vi "AquireTape.vi"(8 "error in (no error)":errorcluster, 10 "Settings":T1={"max velocity"={"Value"=0.0, "Min"=0.0, "Max"=0.0, "StepSize"=0.0, "Tolerance"=0.0, "ValueActual"=0.0}, "continious velocity"={"Value"=0.0, "Min"=0.0, "Max"=0.0, "StepSize"=0.0, "Tolerance"=0.0, "ValueActual"=0.0}, "shake"=enum."off", "direction"=enum."left", "RedRatio"={"Value"=0.0, "Min"=0.0, "Max"=0.0, "StepSize"=0.0, "Tolerance"=0.0, "ValueActual"=0.0}, "StepSize"={"Value"=0.0, "Min"=0.0, "Max"=0.0, "StepSize"=0.0, "Tolerance"=0.0, "ValueActual"=0.0}, "position"={"Value"=0.0, "Min"=0.0, "Max"=0.0, "StepSize"=0.0, "Tolerance"=0.0, "ValueActual"=0.0}, "velocity"={"Value"=0.0, "Min"=0.0, "Max"=0.0, "StepSize"=0.0, "Tolerance"=0.0, "ValueActual"=0.0}, "Step"=enum."off", "Mode"=enum."on demand", "timeout"={"Value"=0.0, "Min"=0.0, "Max"=0.0, "StepSize"=0.0, "Tolerance"=0.0, "ValueActual"=0.0}, "DelayStage"={"Value"=0.0, "Min"=0.0, "Max"=0.0, "StepSize"=0.0, "Tolerance"=0.0, "ValueActual"=0.0}, "TapeMotor"=enum."off", "encoder Axis"=2, "oldpos"=0.0, "ResetEncoder"=enum."off", "tape monitor"=enum."off", "ComPort"="COM1", "Stream Settings"={"My Name"="TapeDrive", "Remote IP Address"="localhost", "Remote Name"="RT"}, "Motor1Axis"={"Value"=0.0, "Min"=0.0, "Max"=0.0, "StepSize"=0.0, "Tolerance"=0.0, "ValueActual"=0.0}, "Motor2Axis"={"Value"=0.0, "Min"=0.0, "Max"=0.0, "StepSize"=0.0, "Tolerance"=0.0, "ValueActual"=0.0}}, 11 "VISA Refnum in":refnum<visa-resource-name>) -> (0 "error out":errorcluster, 1 "RedRatio":dbl, 2 "Settings":T1={"max velocity"={"Value"=0.0, "Min"=0.0, "Max"=0.0, "StepSize"=0.0, "Tolerance"=0.0, "ValueActual"=0.0}, "continious velocity"={"Value"=0.0, "Min"=0.0, "Max"=0.0, "StepSize"=0.0, "Tolerance"=0.0, "ValueActual"=0.0}, "shake"=enum."off", "direction"=enum."left", "RedRatio"={"Value"=0.0, "Min"=0.0, "Max"=0.0, "StepSize"=0.0, "Tolerance"=0.0, "ValueActual"=0.0}, "StepSize"={"Value"=0.0, "Min"=0.0, "Max"=0.0, "StepSize"=0.0, "Tolerance"=0.0, "ValueActual"=0.0}, "position"={"Value"=0.0, "Min"=0.0, "Max"=0.0, "StepSize"=0.0, "Tolerance"=0.0, "ValueActual"=0.0}, "velocity"={"Value"=0.0, "Min"=0.0, "Max"=0.0, "StepSize"=0.0, "Tolerance"=0.0, "ValueActual"=0.0}, "Step"=enum."off", "Mode"=enum."on demand", "timeout"={"Value"=0.0, "Min"=0.0, "Max"=0.0, "StepSize"=0.0, "Tolerance"=0.0, "ValueActual"=0.0}, "DelayStage"={"Value"=0.0, "Min"=0.0, "Max"=0.0, "StepSize"=0.0, "Tolerance"=0.0, "ValueActual"=0.0}, "TapeMotor"=enum."off", "encoder Axis"=2, "oldpos"=0.0, "ResetEncoder"=enum."off", "tape monitor"=enum."off", "ComPort"="COM1", "Stream Settings"={"My Name"="TapeDrive", "Remote IP Address"="localhost", "Remote Name"="RT"}, "Motor1Axis"={"Value"=0.0, "Min"=0.0, "Max"=0.0, "StepSize"=0.0, "Tolerance"=0.0, "ValueActual"=0.0}, "Motor2Axis"={"Value"=0.0, "Min"=0.0, "Max"=0.0, "StepSize"=0.0, "Tolerance"=0.0, "ValueActual"=0.0}}, 3 "VISA Refnum out":refnum<visa-resource-name>, 4 "Position (units)":dbl, 6 "velocity":dbl)   [LabVIEW 2020]
uses:
  settings_TypDef.ctl
  shared/numericVariable_TypeDef.ctl
  shared/OnOffTypeDef.ctl
  Direction_TypDef.ctl
  Mode_TypDEf.ctl
  <vilib>/addons/_JKI.lib/Network_Streams_Connection.llb/PublicSettings.ctl
  shared/CompressAndUpdate(Poly)/CompressAndUpdate(Numeric).vi
  Newport ESP301/Newport ESP301.lvlib
  BaseDriver/BaseDriver.lvclass
  TapeDrive.lvclass
  <vilib>/addons/_JKI.lib/Network_Streams_Connection.llb/NetworkConnection.lvclass
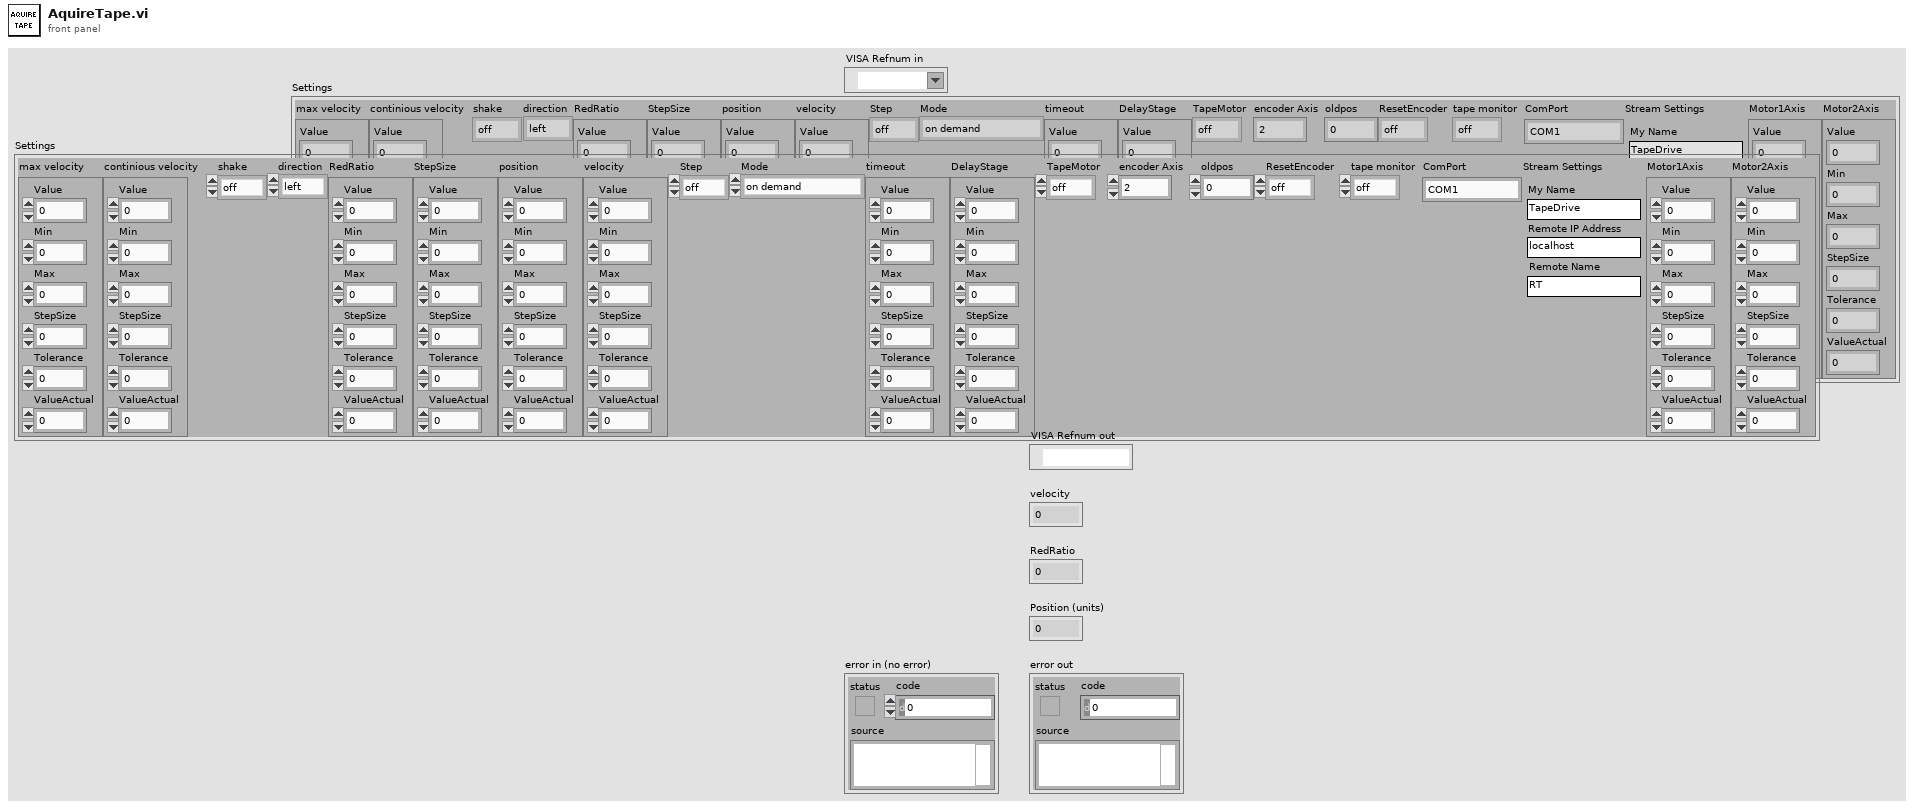
[diagram p1: front panel]
types:
  T1 = typedef "TapeDrive.lvclass/settings_TypDef.ctl" = cluster{"max velocity":T2, "continious velocity":T2, "shake":T3, "direction":T4, "RedRatio":T2, "StepSize":T2, "position":T2, "velocity":T2, "Step":T3, "Mode":T5, "timeout":T2, "DelayStage":T2, "TapeMotor":T3, "encoder Axis":i32, "oldpos":dbl, "ResetEncoder":T3, "tape monitor":T3, "ComPort":string, "Stream Settings":T6, "Motor1Axis":T2, "Motor2Axis":T2}
  T2 = typedef "BaseDriver.lvclass/numericVariable_TypeDef.ctl" = cluster{"Value":dbl, "Min":dbl, "Max":dbl, "StepSize":dbl, "Tolerance":dbl, "ValueActual":dbl}
  T3 = typedef "OnOffTypeDef.ctl" = enum16{"off", "on"}
  T4 = typedef "Direction_TypDef.ctl" = enum16{"left", "right"}
  T5 = typedef "Mode_TypDEf.ctl" = enum16{"on demand", "continuous", "scan"}
  T6 = typedef "NetworkConnection.lvclass/PublicSettings.ctl" = cluster{"My Name":string, "Remote IP Address":string, "Remote Name":string}
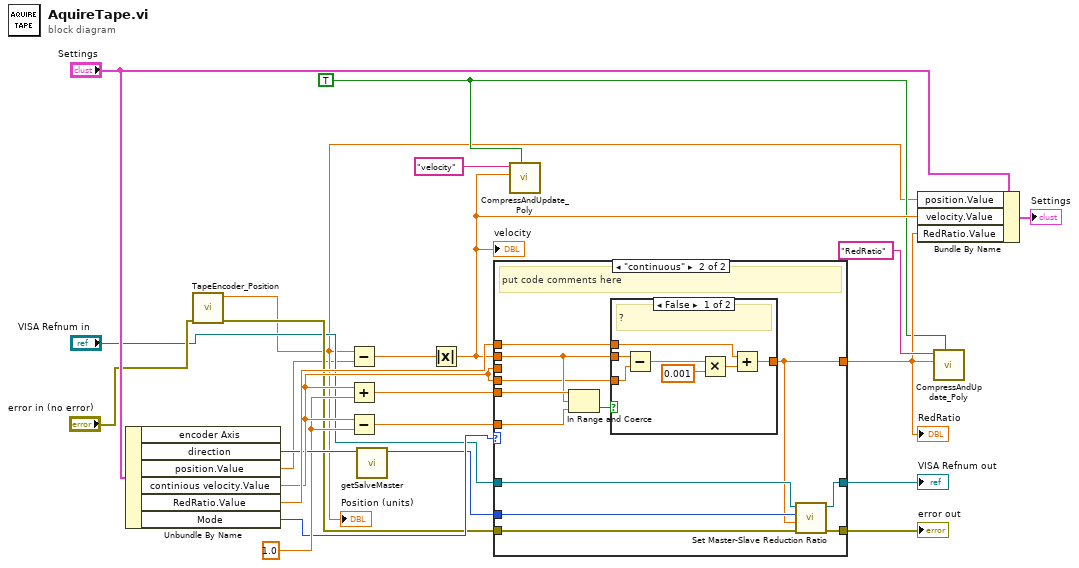
[diagram p0: block diagram]
diagram:
  w8 = TRUE ("force CVT update (false)")
  w16 = 1.0 ("y")
  n1 = Unbundle By Name("Settings") -> ("direction"=w19:T4, "position.Value"=w1:dbl, "continious velocity.Value"=w21:dbl, "RedRatio.Value"=w23:dbl, "Mode"=w7:T5)  [unwired: 1 out]
  n2 = call "TapeEncoder_Position.vi"("error in (no error)"="error in (no error)") -> ("error IO"=w4:errorcluster, "position"=w2:dbl)  [unwired: 9 in]
  "Position (units)" <- w2
  n3 = Subtract(x=w2, y=w1) -> (x-y=w13:dbl)
  n4 = Add(x=w21, y=w16) -> (x+y=w17:dbl)
  n5 = Subtract(x=w21, y=w16) -> (x-y=w18:dbl)
  n6 = call "getSalveMaster.vi"("direction"=w19) -> ("Slave"=w6:i32)  [unwired: 9 in, 1 out]
  n7 = Absolute Value(x=w13) -> (abs(x)=w11:dbl)
  "velocity" <- w11
  n8 = case shown="\"continuous\"" w7 {
    tunnel: "VISA Refnum in" -> [w26 w38]
    tunnel: [w26 w37] -> w14
    tunnel: w4 -> [w25 w36]
    tunnel: [w25 w35] -> w15
    tunnel: w6 -> [_ w34]
    tunnel: w21 -> [_ _]
    tunnel: w11 -> [_ w30]
    tunnel: w17 -> [_ w33]
    tunnel: w18 -> [_ w32]
    tunnel: w21 -> [_ w29]
    tunnel: w23 -> [w24 w28]
    tunnel: [w24 w27] -> w9
    frame "on demand", Default {
    }
    frame "continuous" {
      # "put code comments here"
      n9 = In Range and Coerce(upper limit=w33, x=w30, lower limit=w32) -> (In Range?=w31:bool)  [unwired: 1 out]
      n10 = case shown="False" w31 {
        tunnel: w30 -> [w45 _]
        tunnel: w29 -> [w44 _]
        tunnel: [w40 w46] -> w27
        tunnel: w28 -> [w39 w46]
        frame False {
          # "?"
          n11 = Subtract(x=w45, y=w44) -> (x-y=w43:dbl)
          n12 = Multiply(x=w43, y=0.001) -> (x*y=w41:dbl)
          n13 = Add(x=w39, y=w41) -> (x+y=w40:dbl)
        }
        frame True {
        }
      }
      n14 = call "Set Master-Slave Reduction Ratio.vi"("error in (no error)"=w36, "Reduction Ratio (0)"=w27, "Axis (1)"=w34, "VISA resource name"=w38) -> ("error out"=w35:errorcluster, "VISA resource name out"=w37:refnum<visa-resource-name>)  [unwired: 2 in]
    }
  }
  "RedRatio" <- w9
  "error out" <- w15
  "VISA Refnum out" <- w14
  n15 = call-poly "CompressAndUpdate_Poly.vi"("force CVT update (false)"=w8, "Numeric"=w11, "command or variable name"="velocity") -> ()  [unwired: 8 in, 1 out]
  n16 = Bundle By Name(cluster="Settings", "position.Value"=w2, "velocity.Value"=w11, "RedRatio.Value"=w9) -> (→"Settings":T1)
  n17 = call-poly "CompressAndUpdate_Poly.vi"("force CVT update (false)"=w8, "Numeric"=w9, "command or variable name"="RedRatio") -> ()  [unwired: 8 in, 1 out]
